vi "StreamWrite.vi"(7 "AoType":T1, 8 "error in (no error)":errorcluster, 9 "WavePara":cluster{"Crest":dbl, "Trough":dbl, "Period":dbl}, 10 "Channel":u8, 11 "AIO in":refnum<class "AIO.lvclass">) -> (0 "error out":errorcluster, 3 "AIO out":refnum<class "AIO.lvclass">)   [LabVIEW 2024, in "AIO Actor.lvlib" / "AIO.lvclass"]
uses:
  AIO.lvclass
  AO Type.ctl
  AIO.lvclass/AIO.ctl
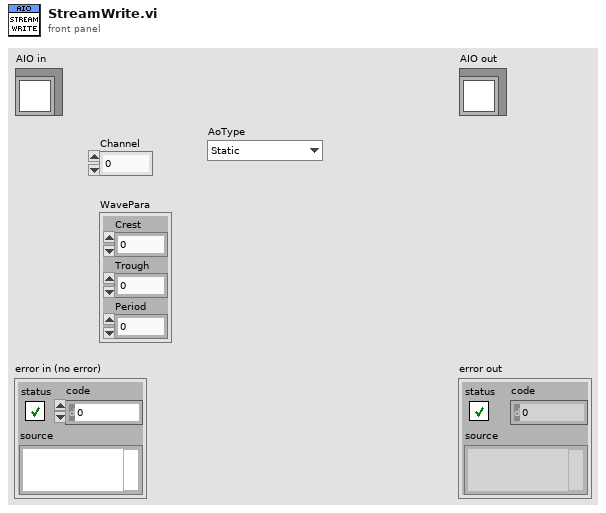
[diagram p1: front panel]
types:
  T1 = typedef "AO Type.ctl" = enum16{"Static", "Streaming", "StopStreaming"}
  T2 = cluster{"AoType":T1, "Channel":u8, "StaticValue":dbl, "WavePara":cluster{"Crest":dbl, "Trough":dbl, "Period":dbl}}
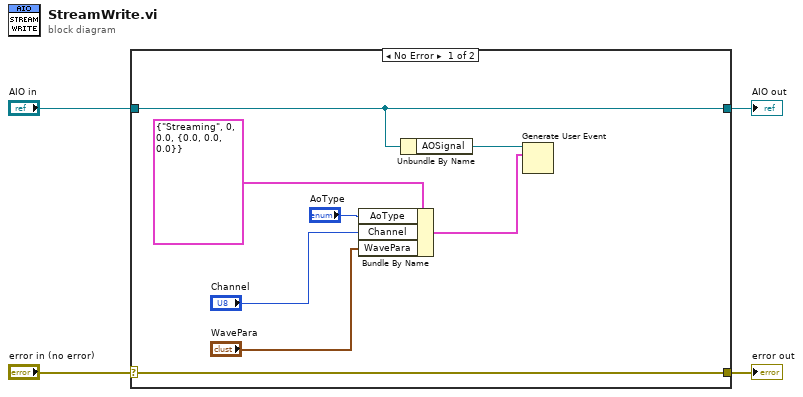
[diagram p0: block diagram]
diagram:
  n1 = case shown="No Error" "error in (no error)" {
    selector: "error in (no error)" -> [w12 w14]
    tunnel: [w12 w14] -> w3
    tunnel: [w11 w13] -> w1
    tunnel: "AIO in" -> [w11 w13]
    frame No Error {
      n2 = Bundle By Name(cluster=T2 {"AoType"=enum."Streaming", "Channel"=0, "StaticValue"=0.0, "WavePara"={"Crest"=0.0, "Trough"=0.0, "Period"=0.0}} ("event data"), "AoType"="AoType", "Channel"="Channel", "WavePara"="WavePara") -> (w6:T2)
      n3 = Unbundle By Name(w11) -> ("AOSignal"=w10:refnum<user-event>)
      n4 = Generate User Event(user event=w10, event data cluster=w6) -> ()  [unwired: 2 in, 2 out]
    }
    frame Error {
    }
  }
  "error out" <- w3
  "AIO out" <- w1
